vi "Modbus Slave Simulator.vi"() -> (0 "error out":errorcluster)   [LabVIEW 2021]
uses:
  File Operations/FGV INI Values Action.ctl
  <vilib>/numeric/Random Number (Range) I64.vi
  <vilib>/numeric/sub_Random U32.vi
  <vilib>/NI/Modbus Library/API/Wrapper/Create TCP Slave.vi
  <vilib>/NI/Modbus Library/API/Slave/Modbus Slave.lvclass
  <vilib>/NI/Modbus Library/API/Wrapper/API Main.lvlib
panel:
  out "Torque Sensor":u16
  out "Termometer":u16(slide) scale=0.0..100.0
  out "Rotation Speed":u16
  out "Elevator Positioning":u16(slide) scale=0.0..10.0
  out "servodriver on/off":bool
  in  "stop":bool
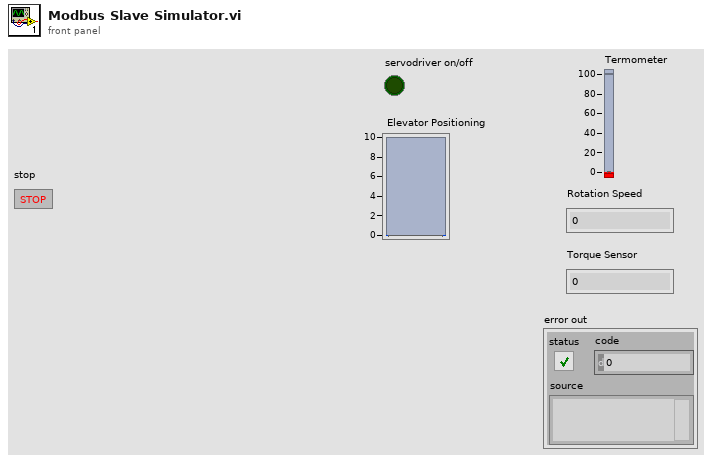
[diagram p1: front panel]
types:
  T1 = cluster{"Session":string, cluster{"Key":string, "value":u32}[]}[]
  T2 = typedef "FGV INI Values Action.ctl" = enum16{"Store", "Get"}
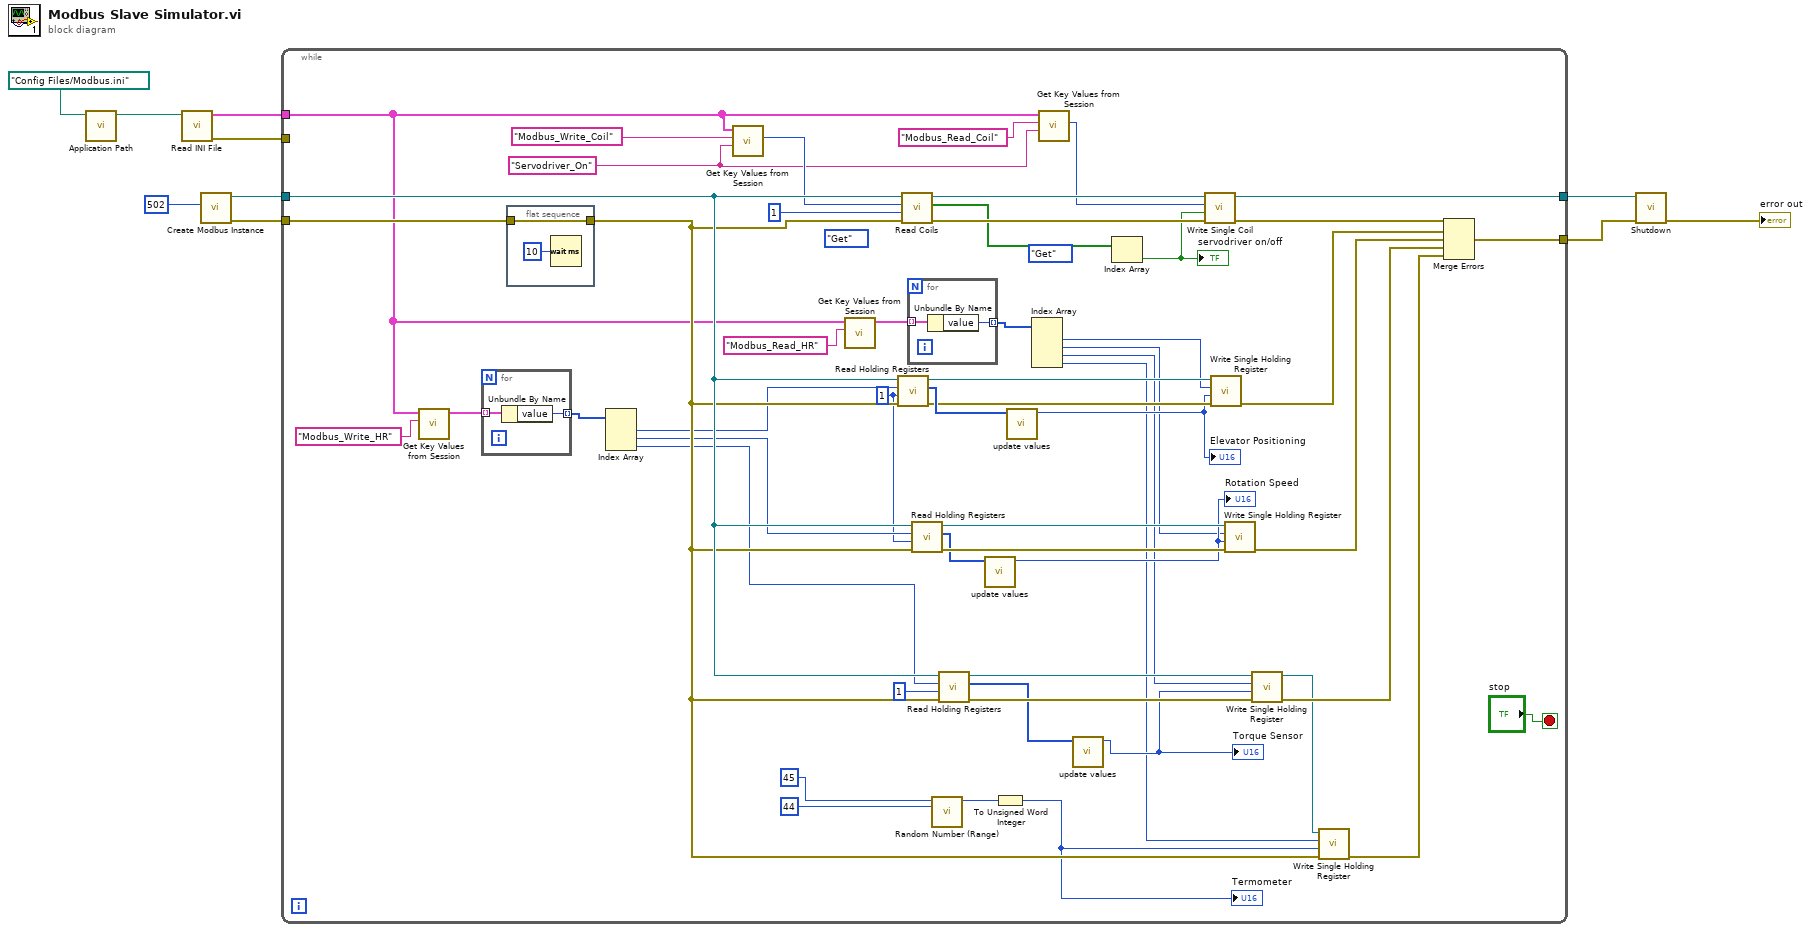
[diagram p0: block diagram]
diagram:
  n1 = call "Application Path.vi"("name or relative path"=path "Config Files/Modbus.ini") -> ("appended path"=w4:path)  [unwired: 10 in]
  n2 = call "Read INI File.vi"("name or relative path"=w4) -> ("error out"=w2:errorcluster, "Ini File"=w1:T1)  [unwired: 9 in]
  n3 = call-poly <vilib>:"Create Modbus Instance.vi"("port (502)"=u16 502) -> ("error out"=w9:errorcluster, "TCP slave instance"=w10:refnum<class "Modbus Slave.lvclass">)  [unwired: 9 in]
  n4 = while {
    tunnel: w10 -> [w45]
    tunnel: w9 -> [w63]
    tunnel: [w54] -> w7
    tunnel: [w51] -> w6
    tunnel: w2 -> [_]
    tunnel: w1 -> [w15]
    stop <- "stop" stop-if-true
    (unwired) FGV_INI_Values_Action."Get" ("FGV Get INI Info")
    (unwired) FGV_INI_Values_Action."Get" ("FGV Get INI Info")
    w26 = "Servodriver_On" ("Key")
    w20 = u16 1 ("number of inputs")
    n5 = call "Get Key Values from Session.vi"("Session"="Modbus_Write_HR", "Ini File"=w15) -> ("Keys Values in Session"=w24:cluster{"Key":string, "value":u32}[])  [unwired: 7 in, 2 out]
    n6 = for {
      tunnel: w24 -> [w68] mode=indexing
      tunnel: [w67] -> w23 mode=indexing
      n7 = Unbundle By Name(w68) -> ("value"=w67:u32)
    }
    n8 = flat-sequence {
      tunnel: w63 -> [w70]
      tunnel: [w70] -> w42
      frame #0 {
        n9 = Wait (ms)(milliseconds to wait=u32 10) -> ()  [unwired: 1 out]
      }
    }
    n10 = Index Array(array=w23) -> (element #1=w22:u32, element #2=w21:u32, element #3=w19:u32)  [unwired: 3 in]
    n11 = call "Get Key Values from Session.vi"("Key"=w26, "Session"="Modbus_Write_Coil", "Ini File"=w15) -> ("Search Key Value"=w29:u32)  [unwired: 6 in, 2 out]
    n12 = call "Get Key Values from Session.vi"("Session"="Modbus_Read_HR", "Ini File"=w15) -> ("Keys Values in Session"=w17:cluster{"Key":string, "value":u32}[])  [unwired: 7 in, 2 out]
    n13 = call-dynamic "Read Holding Registers.vi"("error in"=w42, "number of inputs"=w20, "starting address"=w22, "Modbus slave in"=w45) -> ("error out"=w56:errorcluster, "register values"=w58:u16[], "Modbus slave out"=w57:refnum<class "Modbus Slave.lvclass">)  [unwired: 5 in]
    n14 = call-dynamic "Read Coils.vi"("error in"=w42, "number of inputs"=u16 1, "starting address"=w29, "Modbus slave in"=w45) -> ("error out"=w61:errorcluster, "coils"=w60:bool[], "Modbus slave out"=w62:refnum<class "Modbus Slave.lvclass">)  [unwired: 5 in]
    n15 = for {
      tunnel: w17 -> [w66] mode=indexing
      tunnel: [w65] -> w18 mode=indexing
      n16 = Unbundle By Name(w66) -> ("value"=w65:u32)
    }
    n17 = call-dynamic "Read Holding Registers.vi"("error in"=w42, "number of inputs"=w20, "starting address"=w21, "Modbus slave in"=w45) -> ("error out"=w50:errorcluster, "register values"=w34:u16[], "Modbus slave out"=w49:refnum<class "Modbus Slave.lvclass">)  [unwired: 5 in]
    n18 = call-poly <vilib>:"Random Number (Range).vi"("lower bound (-100)"=i64 44, "upper bound (100)"=i64 45) -> ("number"=w39:i64)  [unwired: 9 in]
    n19 = call-dynamic "Read Holding Registers.vi"("error in"=w42, "number of inputs"=u16 1, "starting address"=w19, "Modbus slave in"=w45) -> ("error out"=w46:errorcluster, "register values"=w32:u16[], "Modbus slave out"=w47:refnum<class "Modbus Slave.lvclass">)  [unwired: 5 in]
    n20 = call "update values.vi"("register values"=w34) -> ("register"=w33:u16)  [unwired: 10 in]
    "Rotation Speed" <- w33
    n21 = To Unsigned Word Integer(number=w39) -> (unsigned 16bit integer=w38:u16)
    "Termometer" <- w38
    n22 = call "update values.vi"("register values"=w58) -> ("register"=w55:u16)  [unwired: 10 in]
    "Elevator Positioning" <- w55
    n23 = Index Array(array=w18) -> (element #1=w14:u32, element #2=w13:u32, element #3=w11:u32, element #4=w12:u32)  [unwired: 4 in]
    n24 = call "Get Key Values from Session.vi"("Key"=w26, "Session"="Modbus_Read_Coil", "Ini File"=w15) -> ("Search Key Value"=w27:u32)  [unwired: 6 in, 2 out]
    n25 = call "update values.vi"("register values"=w32) -> ("register"=w31:u16)  [unwired: 10 in]
    "Torque Sensor" <- w31
    n26 = Index Array(array=w60) -> (element=w59:bool)  [unwired: 1 in]
    "servodriver on/off" <- w59
    n27 = call-dynamic "Write Single Coil.vi"("error in"=w61, "coil to write"=w59, "address"=w27, "Modbus slave in"=w62) -> ("error out"=w53:errorcluster, "Modbus slave out"=w54:refnum<class "Modbus Slave.lvclass">)  [unwired: 6 in]
    n28 = call-dynamic "Write Single Holding Register.vi"("error in"=w56, "register to write"=w55, "address"=w14, "Modbus slave in"=w57) -> ("error out"=w52:errorcluster)  [unwired: 6 in, 1 out]
    n29 = call-dynamic "Write Single Holding Register.vi"("error in"=w50, "register to write"=w33, "address"=w13, "Modbus slave in"=w49) -> ("error out"=w48:errorcluster)  [unwired: 6 in, 1 out]
    n30 = call-dynamic "Write Single Holding Register.vi"("error in"=w46, "register to write"=w31, "address"=w11, "Modbus slave in"=w47) -> ("error out"=w44:errorcluster, "Modbus slave out"=w37:refnum<class "Modbus Slave.lvclass">)  [unwired: 6 in]
    n31 = call-dynamic "Write Single Holding Register.vi"("error in"=w42, "register to write"=w38, "address"=w12, "Modbus slave in"=w37) -> ("error out"=w43:errorcluster)  [unwired: 6 in, 1 out]
    n32 = Merge Errors(w53, w52, w48, w44, w43) -> (w51:errorcluster)
  }
  n33 = call-dynamic "Shutdown.vi"("error in"=w6, "Modbus slave in"=w7) -> ("error out"=→"error out":errorcluster)  [unwired: 9 in]
